vi "create_LED_ramp.vi"(11 "Measurement settings":T1 {"Voltage range" items=["Auto", "200 mV", "2.1 V", "21 V", "210 V"]; "Enable display" items=["False", "True"]; "Auto settling delay" items=["False", "True"]; "Settling delay (ms)" min=0.2 max=999999.9; "Integration time (NPLC)" items=["0.01", "0.1", "1", "10"]; "Current range" items=["Auto", "1 uA", "10 uA", "100 uA", "1 mA", "10 mA", "100 mA", "1 A"]; "Dual JV sweep" items=["False", "True"]; "JV sweep direction" items=["Ascending", "Descending"]; "JV voltage step (V)" min=0.0001 max=5.0 step=0.0001; "Solar cell measurement mode" items=["J-V", "Voc", "Jsc"]; "LED current sweep direction" items=["Ascending", "Descending"]; "LED current sweep mode" items=["Linear", "Logarithmic"]; "Maximum LED Current (A)" min=0.0 max=0.7 step=0.001 format="%#.3f"; "Minimum LED current (A)" min=0.0 max=0.7 step=0.001 format="%#.3f"}) -> (3 "Ramp Pattern":dbl[](array[numeric]))   [LabVIEW 2018]
uses:
  typedefs/measurement_settings.ctl
  <vilib>/Analysis/1siggen.llb/Ramp Pattern by Samples.vi
  <vilib>/Analysis/NI_AALBase.lvlib
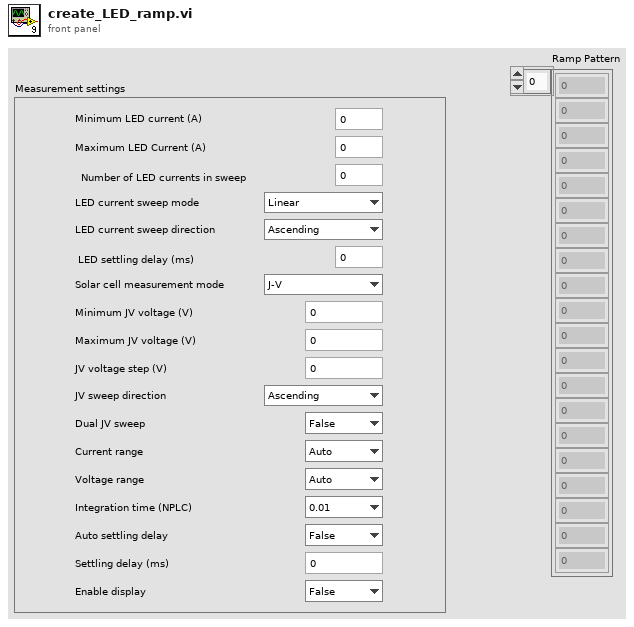
[diagram p1: front panel]
types:
  T1 = typedef "measurement_settings.ctl" = cluster{"Minimum LED current (A)":dbl, "Maximum LED Current (A)":dbl, "Number of LED currents in sweep":u32, "LED current sweep mode":u16, "LED current sweep direction":u16, "LED settling delay (ms)":u32, "Solar cell measurement mode":u16, "Minimum JV voltage (V)":dbl, "Maximum JV voltage (V)":dbl, "JV voltage step (V)":dbl, "JV sweep direction":u16, "Dual JV sweep":u16, "Current range":u16, "Voltage range":u16, "Integration time (NPLC)":u16, "Auto settling delay":u16, "Settling delay (ms)":dbl, "Enable display":u16}
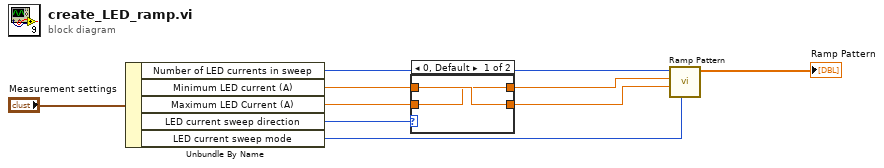
[diagram p0: block diagram]
diagram:
  n1 = Unbundle By Name("Measurement settings") -> ("Number of LED currents in sweep"=w9:u32, "Minimum LED current (A)"=w7:dbl, "Maximum LED Current (A)"=w6:dbl, "LED current sweep direction"=w3:u16, "LED current sweep mode"=w2:u16)
  n2 = case shown="0, Default" w3 {
    tunnel: w7 -> [w11 w13]
    tunnel: w6 -> [w10 w12]
    tunnel: [w10 w13] -> w5
    tunnel: [w11 w12] -> w4
    frame 0, Default {
    }
    frame 1 {
    }
  }
  n3 = call-poly <vilib>:"Ramp Pattern.vi"("type"=w2, "start"=w4, "end"=w5, "samples"=w9) -> ("Ramp Pattern"=→"Ramp Pattern":dbl[])  [unwired: 6 in, 1 out]
